vi "myBeep.vi"(8 "error in (no error)":errorcluster) -> (0 "error out":errorcluster)   [LabVIEW 2017]
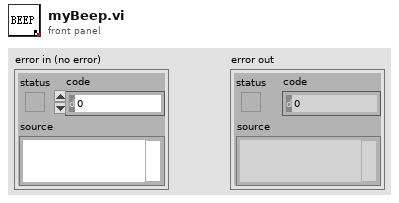
[diagram p1: front panel]
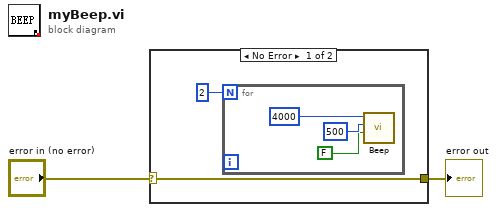
[diagram p0: block diagram]
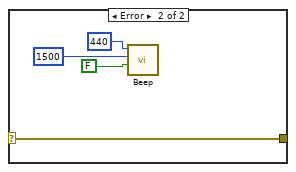
[diagram p2: hidden frame]
diagram:
  n1 = case shown="No Error" "error in (no error)" {
    selector: "error in (no error)" -> [w3 w11]
    tunnel: [w3 w11] -> w1
    frame No Error {
      n2 = for {
        N: 2 -> [_]
        n3 = call <vilib>:"Beep.vi"("use system alert? (T)"=FALSE, "duration (msec)"=u32 500, "frequency (Hz)"=u32 4000) -> ()  [unwired: 9 out]
      }
    }
    frame Error {
      n4 = call <vilib>:"Beep.vi"("use system alert? (T)"=FALSE, "duration (msec)"=u32 1500, "frequency (Hz)"=u32 440) -> ()  [unwired: 9 out]
    }
  }
  "error out" <- w1
